vi "Actor Core.vi"(8 "error in":errorcluster, 11 "MassSpectrumExtractor in":refnum<class "MassSpectrumExtractor.lvclass">) -> (0 "error out":errorcluster, 3 "Actor out":refnum<class "Actor.lvclass">)   [LabVIEW 2014, in "MassSpectrumExtractor.lvclass"]
doc: "(<B>Filename</B>: Actor Framework.lvlib:Actor.lvclass:Actor Core.vi)\n\nReceives messages to the actor, reacts to them, and initiates any error handling that may shut the actor down.\n\nDescendant classes may override this VI to append parallel tasks for the actor to complete while it handles messages. Overrides use the Call Parent Method node."
uses:
  MassSpectrumExtractor.lvclass
  <vilib>/ActorFramework/Actor/Actor.lvclass
  Graph with cursors/Graph with cursors XControl.xctl
  MassSpectrumExtractor.lvclass/MassSpectrumExtractor.ctl
  <vilib>/ActorFramework/Actor/Actor.lvclass/Actor.ctl
  <vilib>/ActorFramework/Message Enqueuer/Message Enqueuer.lvclass/Message Enqueuer.ctl
  Framework/Model/Data/Data1D/Data1D.lvclass
  <vilib>/ActorFramework/Message Enqueuer/Init from Existing Queue.vi
  <vilib>/ActorFramework/Message Enqueuer/Message Enqueuer.lvclass
  Framework/Extractor/AbstractExtractor1D/AbstractExtractor1D.lvclass
  Framework/Interfaces/Viewable Actor/Viewable Actor.lvclass
  Framework/Interfaces/Observable Actor/Observable Actor.lvclass
panel:
  in  "Clear":bool
  out "IntegralArray":cluster{"Array":dbl[], "Array":dbl[]}[](array[cluster])
  out "MaximumArray":cluster{"Array":dbl[], "Array":dbl[]}[](array[cluster])
  in  "Tab Control":enum32{"Integral", "Maximum"}(tab)
  out "IntegralGraph":cluster{"X":dbl[], "Y":dbl[]}[](graph)
  out "MaximumGraph":cluster{"X":dbl[], "Y":dbl[]}[](graph)
  out "Graph":waveform(dbl)(xcontrol)
  out "Stop":bool=TRUE
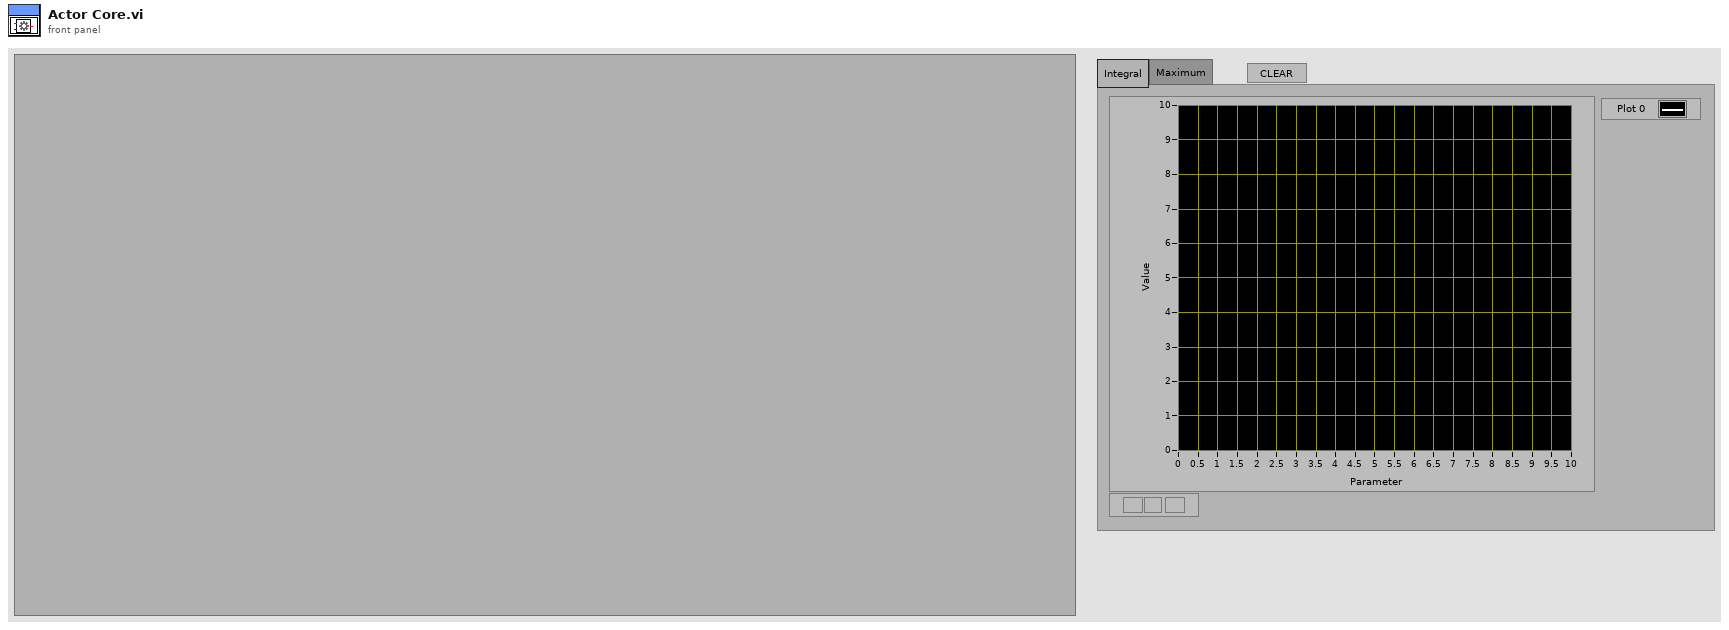
[diagram p1: front panel]
types:
  T1 = cluster{"Result Graph":refnum<vi>, "Input Graph":refnum<vi>}
  T2 = typedef "Observable Actor.lvlib/Observable Actor.lvclass/Observer.ctl" = refnum<queue>
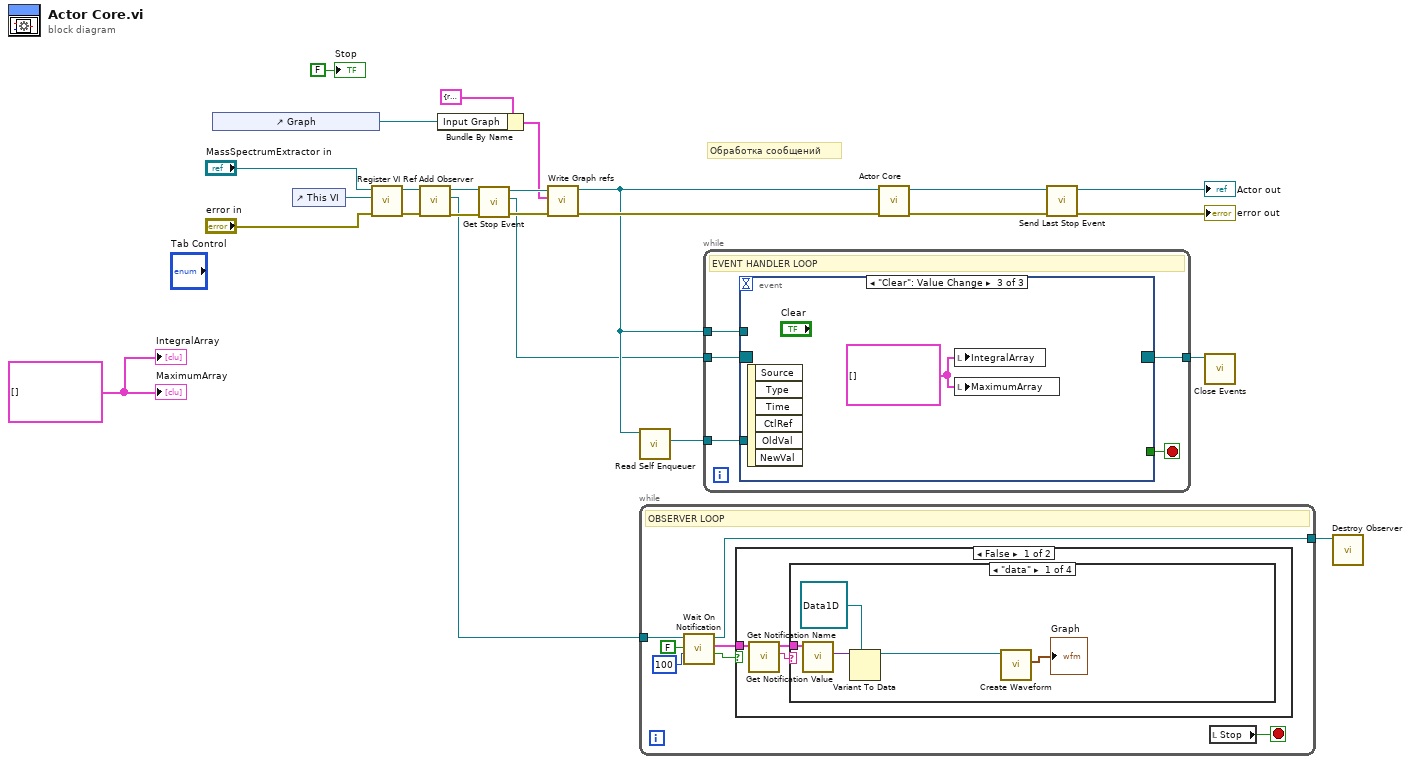
[diagram p0: block diagram]
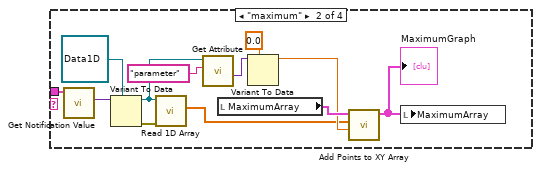
[diagram p2: hidden frame]
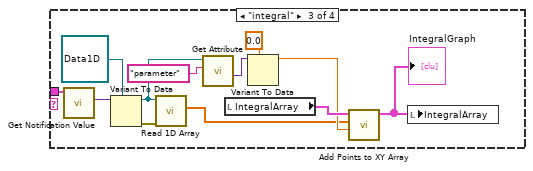
[diagram p3: hidden frame]
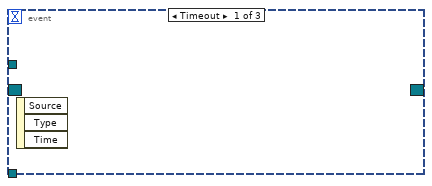
[diagram p6: hidden frame]
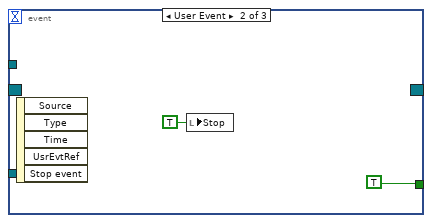
[diagram p7: hidden frame]
diagram:
  w1 = cluster{dbl[], dbl[]}[] []
  # "Обработка сообщений"
  n1 = control-ref of="Graph"() -> (w2:refnum<vi>)
  n2 = control-ref of="This VI"() -> (w25:refnum<vi>)
  n3 = call "Register VI Ref.vi"("error in (no error)"="error in", "VI ref"=w25, "Viewable Actor in"="MassSpectrumExtractor in") -> ("error out"=w10:errorcluster, "Viewable Actor out"=w11:refnum<class "MassSpectrumExtractor.lvclass">)  [unwired: 7 in]
  n4 = call-dynamic "Add Observer.vi"("error in (no error)"=w10, "Observable Actor in"=w11) -> ("error out"=w12:errorcluster, "new observer"=w5:T2, "Observable Actor out"=w13:refnum<class "MassSpectrumExtractor.lvclass">)  [unwired: 7 in]
  n5 = Bundle By Name(cluster=T1 {"Result Graph"=refnum, "Input Graph"=refnum} ("Graph refs"), "Input Graph"=w2) -> (w3:T1)
  n6 = call-dynamic "Get Stop Event.vi"("error in (no error)"=w12, "Observable Actor in"=w13) -> ("error out"=w8:errorcluster, "Events"=w7:refnum<event-registration>, "Observable Actor out"=w9:refnum<class "MassSpectrumExtractor.lvclass">)  [unwired: 7 in]
  n7 = call "Write Graph refs.vi"("error in (no error)"=w8, "Graph refs"=w3, "MassSpectrumExtractor in"=w9) -> ("error out"=w20:errorcluster, "MassSpectrumExtractor out"=w19:refnum<class "MassSpectrumExtractor.lvclass">)  [unwired: 7 in]
  n8 = call <vilib>:"Read Self Enqueuer.vi"("Actor"=w19) -> ("Self Enqueuer"=w22:refnum<class "Message Enqueuer.lvclass">)  [unwired: 10 in]
  n9 = while {
    tunnel: w5 -> [w26]
    tunnel: [w29] -> w6
    stop <- w32 stop-if-true
    # "OBSERVER LOOP"
    n10 = call "Wait On Notification.vi"("timeout in ms (-1)"=100, "ignore previous (F)"=FALSE, "observer in"=w26) -> ("timed out?"=w27:bool, "notification"=w28:cluster{"value":variant, "name":string}, "observer out"=w29:T2)  [unwired: 5 in, 1 out]
    n11 = case shown="False" w27 {
      tunnel: w28 -> [w35 _]
      frame False {
        n12 = call "Get Notification Name.vi"("notification in"=w35) -> ("name"=w33:string, "notification out"=w34:cluster{"value":variant, "name":string})  [unwired: 9 in]
        n13 = case shown="\"data\"" w33 {
          tunnel: w34 -> [w39 w51 w63 _]
          frame "data" {
            n14 = call "Get Notification Value.vi"("notification in"=w39) -> ("data"=w40:variant)  [unwired: 7 in, 1 out]
            n15 = Variant To Data(type=refnum<class "Data1D.lvclass"> refnum ("Data1D in"), Variant=w40) -> (data=w36:refnum<class "Data1D.lvclass">)  [unwired: 1 in, 1 out]
            n16 = call "Create Waveform.vi"("Data1D in"=w36) -> ("Waveform"=→"Graph":waveform(dbl))  [unwired: 8 in, 2 out]
          }
          frame "maximum" {
            n17 = call "Get Notification Value.vi"("notification in"=w51) -> ("data"=w52:variant)  [unwired: 7 in, 1 out]
            n18 = Variant To Data(type=refnum<class "Data1D.lvclass"> refnum ("Data1D in"), Variant=w52) -> (data=w41:refnum<class "Data1D.lvclass">, error out=w50:errorcluster)  [unwired: 1 in]
            n19 = call "Read 1D Array.vi"("error in (no error)"=w50, "Data1D in"=w41) -> ("1D Array"=w43:dbl[])  [unwired: 7 in, 2 out]
            n20 = call-dynamic "Get Attribute.vi"("Name"="parameter", "AbstractData in"=w41) -> ("value"=w47:variant)  [unwired: 6 in, 3 out]
            n21 = local read "MaximumArray"() -> (w45:cluster{"Array":dbl[], "Array":dbl[]}[])
            n22 = Variant To Data(type=0.0, Variant=w47) -> (data=w44:dbl)  [unwired: 1 in, 1 out]
            n23 = call "Add Points to XY Array.vi"("Parameter"=w44, "Values"=w43, "Array in"=w45) -> ("Array out"=w42:cluster{"X":dbl[], "Y":dbl[]}[])  [unwired: 8 in]
            "MaximumGraph" <- w42
            n24 = local write "MaximumArray"(w42) -> ()
          }
          frame "integral" {
            n25 = call "Get Notification Value.vi"("notification in"=w63) -> ("data"=w64:variant)  [unwired: 7 in, 1 out]
            n26 = Variant To Data(type=refnum<class "Data1D.lvclass"> refnum ("Data1D in"), Variant=w64) -> (data=w53:refnum<class "Data1D.lvclass">, error out=w62:errorcluster)  [unwired: 1 in]
            n27 = call "Read 1D Array.vi"("error in (no error)"=w62, "Data1D in"=w53) -> ("1D Array"=w55:dbl[])  [unwired: 7 in, 2 out]
            n28 = call-dynamic "Get Attribute.vi"("Name"="parameter", "AbstractData in"=w53) -> ("value"=w59:variant)  [unwired: 6 in, 3 out]
            n29 = local read "IntegralArray"() -> (w57:cluster{"Array":dbl[], "Array":dbl[]}[])
            n30 = Variant To Data(type=0.0, Variant=w59) -> (data=w56:dbl)  [unwired: 1 in, 1 out]
            n31 = call "Add Points to XY Array.vi"("Parameter"=w56, "Values"=w55, "Array in"=w57) -> ("Array out"=w54:cluster{"X":dbl[], "Y":dbl[]}[])  [unwired: 8 in]
            "IntegralGraph" <- w54
            n32 = local write "IntegralArray"(w54) -> ()
          }
          frame Default {
          }
        }
      }
      frame True {
      }
    }
    n33 = local read "Stop"() -> (w32:bool)
  }
  n34 = while {
    tunnel: w7 -> [w69]
    tunnel: w22 -> [w68]
    tunnel: [w67] -> w14
    tunnel: w19 -> [w65]
    stop <- w66 stop-if-true
    # "EVENT HANDLER LOOP"
    n35 = event shown="[2] \"Clear\": Value Change" {
      selector: w69 -> [_ _ _]
      dyn-events: [_ _ _] -> w67
      timeout: _ -> [_ _ _]
      tunnel: w68 -> [_ _ _]
      tunnel: [_ TRUE _] -> w66
      tunnel: w65 -> [_ _ _]
      event Timeout {
        n36 = event-data() -> ()  [unwired: 1 in, 3 out]
      }
      event User Event {
        n37 = event-data() -> ()  [unwired: 1 in, 5 out]
        n38 = local write "Stop"(TRUE ("Stop")) -> ()
      }
      event "Clear": Value Change {
        w72 = cluster{dbl[], dbl[]}[] []
        n39 = event-data() -> ()  [unwired: 1 in, 6 out]
        n40 = local write "IntegralArray"(w72) -> ()
        n41 = local write "MaximumArray"(w72) -> ()
      }
    }
  }
  n42 = call-parent "Actor Core.vi"("error in"=w20, "Actor in"=w19) -> ("error out"=w17:errorcluster, "Actor out"=w18:refnum<class "Actor.lvclass">)  [unwired: 8 in]
  n43 = call "Send Last Stop Event.vi"("error in (no error)"=w17, "Actor in"=w18) -> ("error out"=→"error out":errorcluster, "Actor  out"=→"Actor out":refnum<class "Actor.lvclass">)  [unwired: 8 in]
  n44 = call "Close Events.vi"("events"=w14) -> ()  [unwired: 11 in]
  n45 = call "Destroy Observer.vi"("observer in"=w6) -> ()  [unwired: 11 in]
  "Stop" <- FALSE ("Stop")
  "MaximumArray" <- w1
  "IntegralArray" <- w1
